vi "VICloseSave.vi"(8 "error in (no error)":errorcluster, 11 "VI in":refnum<vi>) -> (0 "error out":errorcluster)   [LabVIEW 2013]
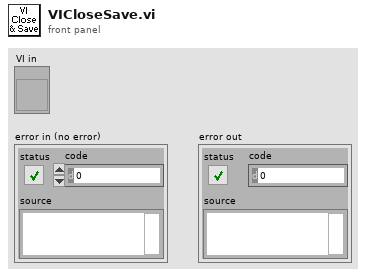
[diagram p1: front panel]
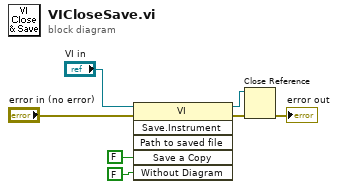
[diagram p0: block diagram]
diagram:
  n1 = invoke class="VI" method="Save.Instrument"(reference="VI in", error in="error in (no error)", "Save a Copy"=FALSE, "Without Diagram"=FALSE) -> (reference out=w7:refnum<vi>, error out=w6:errorcluster)  [unwired: 2 in, 4 out]
  n2 = Close Reference(reference=w7, error in (no error)=w6) -> (error out=→"error out":errorcluster)
